vi "GyroRxLoop.vi"   [LabVIEW 2016]
uses:
  GyroRxLoopData.ctl
  GyroRxLoopStates.ctl
  GyroSBITSample.ctl
  GyroLBITSample.ctl
  GyroSample.ctl
  GyroErrorSample.ctl
  GyroErrorCodes.ctl
  <vilib>/Platform/TimedLoop/XDataNode/timing_clust.ctl
  <vilib>/Platform/TimedLoop/XDataNode/nitl_modes.ctl
  <vilib>/Platform/TimedLoop/XDataNode/wakeup.ctl
  <vilib>/rvi/Emulation/niFpgaSctlEmulationGetInTimedLoop.vi
  <vilib>/rvi/Emulation/niFpgaEmulationReportErrorSimple.vi
  <vilib>/rvi/Emulation/niFpgaGetClockAttributes.vi
  <vilib>/rvi/Emulation/niFpgaCriticalErrorInLSC.vi
  <vilib>/rvi/Emulation/niFpgaEmulationIsFPGAContextNoSignature.vi
  <vilib>/rvi/errors/niFpgaSetErrorForExecOnDevCompSimple.vi
  <vilib>/rvi/eio/common/nirviEmuReportErrorAndStop.vi
  <vilib>/rvi/DataTransferAndStorage/Container/Common/niFpgaContainerGetUniqueNameForEmu.vi
  <vilib>/rvi/FIFO/Fifo_Resource/nirvififoEmulationSetSize.vi
  <vilib>/rvi/FIFO/Fifo_Resource/nirviFifoEmulationQueueMgr.vi
  <instcachedir>/0/nirviFifoEmulationQueueMgr_E5CAEC123FF24DC58D834DCA3CDAA9B5.lvgen/nirviFifoEmulationQueueMgr_E5CAEC123FF24DC58D834DCA3CDAA9B5_009.vi
  <vilib>/Utility/error.llb/Clear Errors.vi
  <vilib>/rvi/FIFO/Fifo_Resource/nirvififoEmulationCreateLock.vi
  <vilib>/rvi/Emulation/niFpgaProcessEmulError.vi
  <vilib>/rvi/FIFO/Fifo_Resource/nirvififoEmulationObtainLock.vi
  <vilib>/rvi/FIFO/Fifo_Resource/nirvififoEmulationReleaseLock.vi
  <vilib>/rvi/occurrence/nirviWaitOnOccurrenceBase.vi
  <vilib>/rvi/errors/nirviReportUnexpectedCaseInternalError.vi
  <vilib>/rvi/errors/nirviReportUnexpectedCaseInternalError (U32).vi
  <vilib>/rvi/FIFO/Fifo_Resource/nirvififoEmulationDetermineInputValidOut.vi
  <vilib>/rvi/Memory/Memory_Emulation/niFpgaMemoryEmulationCacheClearOnFirstRun.vi
  <vilib>/rvi/Memory/Memory_Emulation/nirvimemoryEmulationManagerCache_MakeExclusive.vi
  <vilib>/rvi/Memory/Memory_Emulation/niFpgaMemoryEmulationValidateCache.vi
  <vilib>/rvi/Memory/Memory_Emulation/nirvimemoryEmulationManagerCache_InsertValue.vi
  <vilib>/rvi/Memory/Memory_Emulation/nirvimemoryEmulationManagerCache_ReleaseExclusive.vi
  <vilib>/rvi/Memory/Memory_Emulation/nirvimemoryEmulationManagerCache_GetValue.vi
  <vilib>/rvi/Memory/Memory_Emulation/nirvimemoryEmulationManagerCache_SetValue.vi
  <instcachedir>/0/nirviFifoEmulationQueueMgr_E5CAEC123FF24DC58D834DCA3CDAA9B5.lvgen/nirviFifoEmulationQueueMgr_E5CAEC123FF24DC58D834DCA3CDAA9B5_040.vi
  <instcachedir>/0/nirviFifoEmulationQueueMgr_E5CAEC123FF24DC58D834DCA3CDAA9B5.lvgen/nirviFifoEmulationQueueMgr_E5CAEC123FF24DC58D834DCA3CDAA9B5_041.vi
  <instcachedir>/0/nirviFifoEmulationQueueMgr_E5CAEC123FF24DC58D834DCA3CDAA9B5.lvgen/nirviFifoEmulationQueueMgr_E5CAEC123FF24DC58D834DCA3CDAA9B5_004.vi
  <instcachedir>/0/nirviFifoEmulationQueueMgr_E5CAEC123FF24DC58D834DCA3CDAA9B5.lvgen/nirviFifoEmulationQueueMgr_E5CAEC123FF24DC58D834DCA3CDAA9B5_006.vi
  <instcachedir>/0/nirviFifoEmulationQueueMgr_E5CAEC123FF24DC58D834DCA3CDAA9B5.lvgen/nirviFifoEmulationQueueMgr_E5CAEC123FF24DC58D834DCA3CDAA9B5_042.vi
  <instcachedir>/0/nirviFifoEmulationQueueMgr_E5CAEC123FF24DC58D834DCA3CDAA9B5.lvgen/nirviFifoEmulationQueueMgr_E5CAEC123FF24DC58D834DCA3CDAA9B5_043.vi
  <vilib>/Platform/TimedLoop/XDataNode/XDataNode.xnode
  <vilib>/rvi/DataTransferAndStorage/Container/XNode/niFpgaContainer.xnode
  <vilib>/rvi/FIFO/Fifo_Resource/nirvififoEmulationRead.vi
  <vilib>/rvi/FIFO/Fifo_Resource/nirvififoEmulationWrite.vi
  <vilib>/rvi/DataTransferAndStorage/Register/Emulation/niFpgaRegisterEmulation.vi
  <vilib>/Platform/TimedLoop/XDataNode/XDNodeRunTimeDep.lvlib
types:
  T1 = typedef "GyroRxLoopData.ctl" = cluster{"State":T2, "Timestamp":u64, "Timeout":i32, "CRC":u32, "Checksum":u8, "IsLBIT":bool, "ReservedCount":u8, "SBITSample":T3, "LBITSample":T4, "Sample":T5, "ErrorSample":T6}
  T2 = typedef "GyroRxLoopStates.ctl" = enum16{"ReadHeader3", "IgnoreASCIIResponse", "ReadNormalHeader2", "ReadNormalHeader1", "ReadBITHeader0", "ReadBIT0", "ReadBIT1", "ReadBIT2", "ReadBIT3", "ReadBIT4", "ReadBIT5", "ReadBIT6", "ReadBIT7", "ReadChecksum", "PrepareSBIT", "MoveSBIT", "PrepareLBIT", "MoveLBIT", "ReadSampleHeader0", "ReadSampleX3", "ReadSampleX2", "ReadSampleX1", "ReadSampleX0", "ReadSampleY3", "ReadSampleY2", "ReadSampleY1", "ReadSampleY0", "ReadSampleZ3", "ReadSampleZ2", "ReadSampleZ1", "ReadSampleZ0", "ReadSampleReserved", "ReadSampleStatus", "ReadSampleSequenceNumber", "ReadSampleTemperature1", "ReadSampleTemperature0", "ReadSampleCRC3", "ReadSampleCRC2", "ReadSampleCRC1", "ReadSampleCRC0", "VerifyCRC", "PrepareSample", "MoveSample", "ResponseHeaderError", "ResponseCRCError", "ResponseTimeoutError", "ResponseChecksumError", "PrepareErrorCode", "MoveErrorCode", "ClearCRC", "WaitForCRCCleared"}
  T3 = typedef "GyroSBITSample.ctl" = cluster{"Timestamp":u64, "TxBytes":u64, "RxBytes":u64, "TxFrames":u64, "RxFrames":u64, "BIT0":u8, "BIT1":u8, "BIT2":u8, "BIT3":u8, "BIT4":u8, "BIT5":u8}
  T4 = typedef "GyroLBITSample.ctl" = cluster{"Timestamp":u64, "TxBytes":u64, "RxBytes":u64, "TxFrames":u64, "RxFrames":u64, "BIT0":u8, "BIT1":u8, "BIT2":u8, "BIT3":u8, "BIT4":u8, "BIT5":u8, "BIT6":u8, "BIT7":u8}
  T5 = typedef "GyroSample.ctl" = cluster{"Timestamp":u64, "TxBytes":u64, "RxBytes":u64, "TxFrames":u64, "RxFrames":u64, "GyroX":u32, "GyroY":u32, "GyroZ":u32, "Status":u8, "SequenceNumber":u8, "Temperature":i16}
  T6 = typedef "GyroErrorSample.ctl" = cluster{"Timestamp":u64, "TxBytes":u64, "RxBytes":u64, "TxFrames":u64, "RxFrames":u64, "ErrorCode":T7}
  T7 = typedef "GyroErrorCodes.ctl" = enum8{"None", "ResponseHeaderError", "ResponseCRCError", "ResponseTimeoutError", "ResponseChecksumError"}
  T8 = typedef "XDNodeRunTimeDep.lvlib/timing_clust.ctl" = cluster{"Expected End [f-1]":u64, "Actual End [f-1]":u64, "Finished Late? [f-1]":bool, "Expected End [i-1]":u64, "Actual End [i-1]":u64, "Finished Late? [i-1]":bool, "Expected Start [i]":u64, "Actual Start [i]":u64, "Expected Start [f]":u64, "Actual Start [f]":u64, "Source Name":string, "Structure Name":string, "Period":i64, "Deadline":i64, "Offset":i64, "Start":i64, "Priority":i32, "Timeout":i32, "Mode":T9, "Wakeup Reason":T10, "Error":errorcluster, "Source Type":string, "Secondary Source Type":string, "Global End Time":u64, "Global Start Time":u64, "Frame Duration":u64, "Iteration Duration":u64, "Assigned CPU":i32, "I/O Scan Engine Mode":u32}
  T9 = typedef "XDNodeRunTimeDep.lvlib/nitl_modes.ctl" = enum32{"No Change", "Process missed periods, maintain original phase", "Discard missed periods, maintain original phase", "Process missed periods, ignore original phase", "Discard missed periods, ignore original phase"}
  T10 = typedef "XDNodeRunTimeDep.lvlib/wakeup.ctl" = enum32{"Normal", "Aborted", "Asynchronous wakeup", "Timing source error", "Timed loop error", "Timeout"}
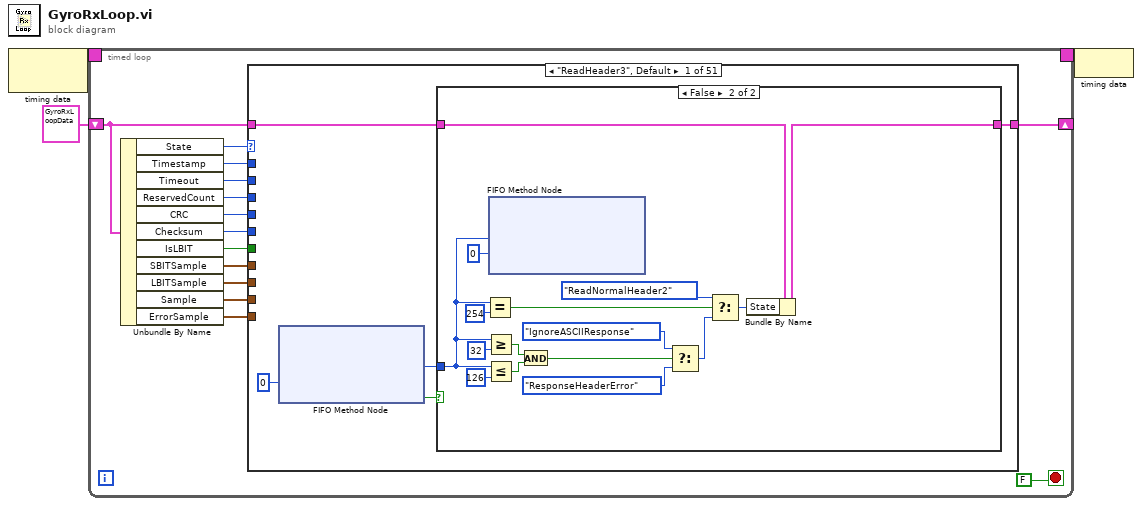
[diagram p0: block diagram]
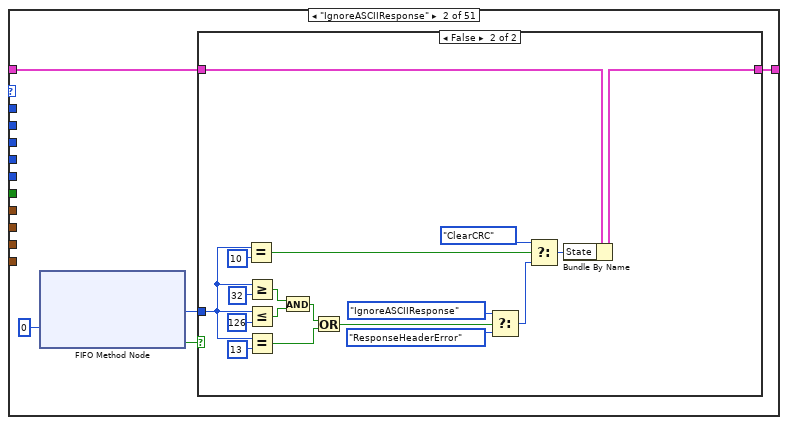
[diagram p3: hidden frame]
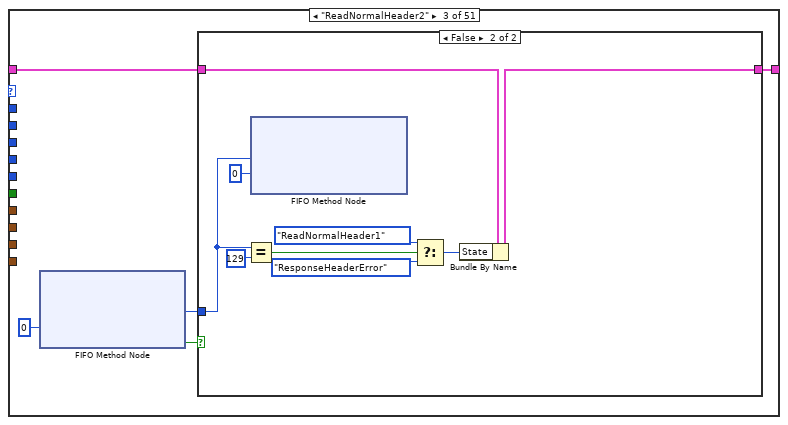
[diagram p5: hidden frame]
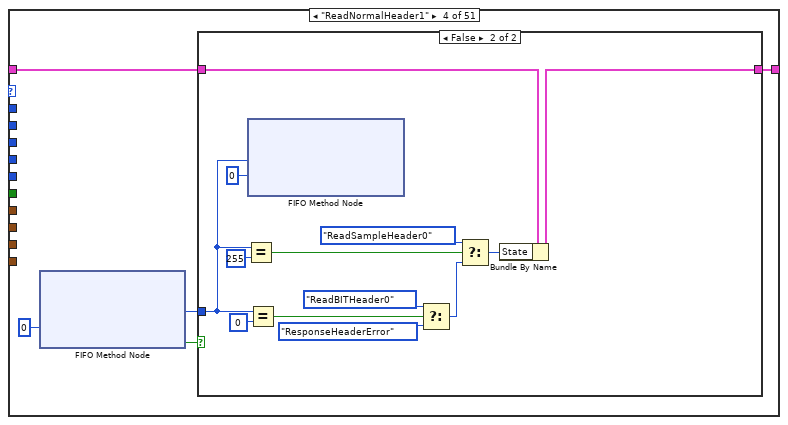
[diagram p7: hidden frame]
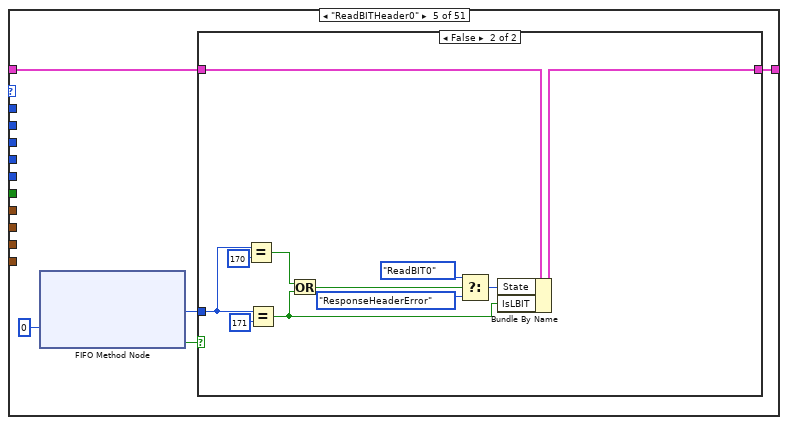
[diagram p9: hidden frame]
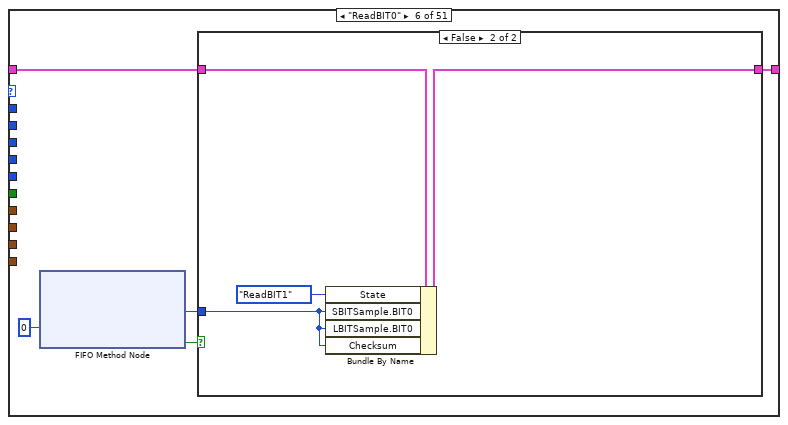
[diagram p11: hidden frame]
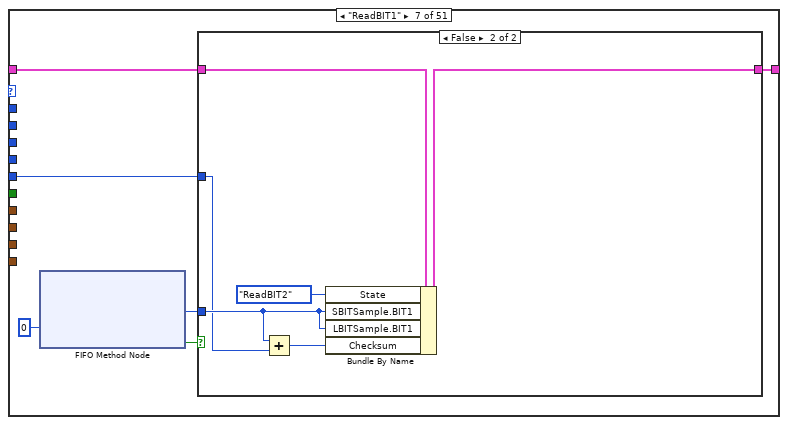
[diagram p13: hidden frame]
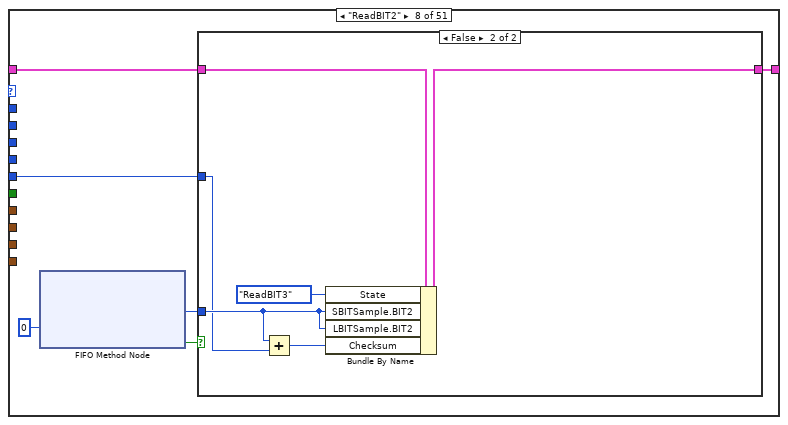
[diagram p15: hidden frame]
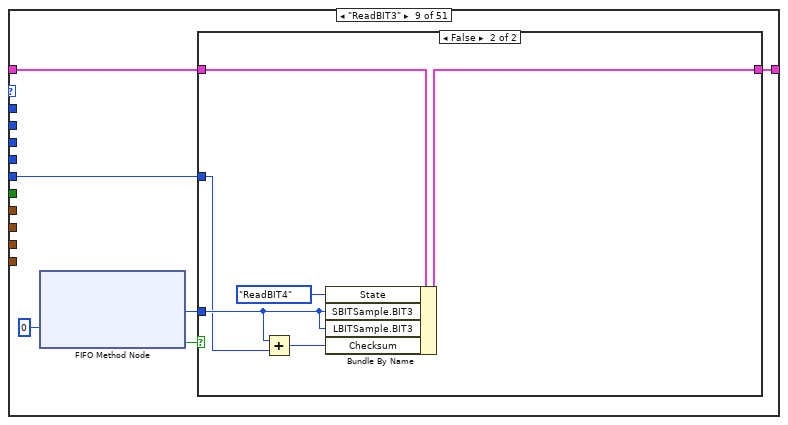
[diagram p17: hidden frame]
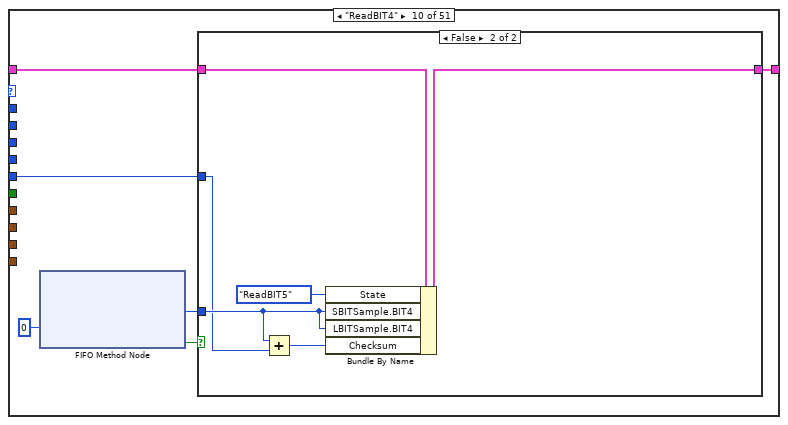
[diagram p19: hidden frame]
diagram:
  n1 = node-c288() -> (w3:T8)  [unwired: 1 in]
  n2 = timed-loop {
    timing: w3 -> [_]
    timing-out: [_] -> w2
    shift-right: [w17] -> _
    shift-left: T1 {"State"=enum."ReadHeader3", "Timestamp"=0, "Timeout"=0, "CRC"=0, "Checksum"=0, "IsLBIT"=FALSE, "ReservedCount"=0, "SBITSample"={"Timestamp"=0, "TxBytes"=0, "RxBytes"=0, "TxFrames"=0, "RxFrames"=0, "BIT0"=0, "BIT1"=0, "BIT2"=0, "BIT3"=0, "BIT4"=0, "BIT5"=0}, "LBITSample"={"Timestamp"=0, "TxBytes"=0, "RxBytes"=0, "TxFrames"=0, "RxFrames"=0, "BIT0"=0, "BIT1"=0, "BIT2"=0, "BIT3"=0, "BIT4"=0, "BIT5"=0, "BIT6"=0, "BIT7"=0}, "Sample"={"Timestamp"=0, "TxBytes"=0, "RxBytes"=0, "TxFrames"=0, "RxFrames"=0, "GyroX"=0, "GyroY"=0, "GyroZ"=0, "Status"=0, "SequenceNumber"=0, "Temperature"=0}, "ErrorSample"={"Timestamp"=0, "TxBytes"=0, "RxBytes"=0, "TxFrames"=0, "RxFrames"=0, "ErrorCode"=enum."None"}} ("GyroRxLoopData") -> [w16]
    stop <- FALSE stop-if-true
    n3 = Unbundle By Name(w16) -> ("State"=w15:T2, "Timestamp"=w14:u64, "Timeout"=w13:i32, "ReservedCount"=w9:u8, "CRC"=w12:u32, "Checksum"=w11:u8, "IsLBIT"=w10:bool, "SBITSample"=w8:T3, "LBITSample"=w7:T4, "Sample"=w6:T5, "ErrorSample"=w5:T6)
    n4 = case shown="\"ReadHeader3\", Default" w15 {
      tunnel: [w18 w40 w64 w79 w98 w115 w126 w139 w152 w165 w179 w195 w208 w222 w245 w250 w258 w263 w265 w280 w294 w310 w326 w340 w354 w370 w386 w400 w414 w430 w446 w462 w479 w490 w501 w515 w529 w545 w561 w577 w591 w611 w616 w620 w624 w628 w632 w640 w645 w650 w657] -> w17
      tunnel: w16 -> [w19 w41 w65 w80 w99 w116 w127 w140 w153 w166 w180 w196 w209 w223 w246 w251 w259 w264 w266 w281 w295 w311 w327 w341 w355 w371 w387 w401 w415 w431 w447 w463 w480 w491 w502 w516 w530 w546 w562 w578 w592 w612 w617 w621 w625 w629 w633 w641 w646 w651 w658]
      tunnel: w14 -> [_ _ _ _ _ _ _ _ _ _ _ _ _ _ w243 _ w256 _ _ _ _ _ _ _ _ _ _ _ _ _ _ _ _ _ _ _ _ _ _ _ _ w609 _ _ _ _ _ w638 _ _ _]
      tunnel: w13 -> [_ _ _ _ _ _ _ _ _ _ _ _ _ _ _ _ _ _ _ _ _ _ _ _ _ _ _ _ _ _ _ _ _ _ _ _ _ _ _ _ _ _ _ _ _ _ _ _ _ _ _]
      tunnel: w12 -> [_ _ _ _ _ _ _ _ _ _ _ _ _ _ _ _ _ _ _ _ _ _ _ _ _ _ _ _ _ _ _ _ _ _ _ _ _ w544 w560 w576 w590 _ _ _ _ _ _ _ _ _ _]
      tunnel: w11 -> [_ _ _ _ _ _ w125 w138 w151 w164 w178 w194 w207 w221 _ _ _ _ _ _ _ _ _ _ _ _ _ _ _ _ _ _ _ _ _ _ _ _ _ _ _ _ _ _ _ _ _ _ _ _ _]
      tunnel: w10 -> [_ _ _ _ _ _ _ _ _ _ w177 _ _ w220 _ _ _ _ _ _ _ _ _ _ _ _ _ _ _ _ _ _ _ _ _ _ _ _ _ _ _ _ _ _ _ _ _ _ _ _ _]
      tunnel: w9 -> [_ _ _ _ _ _ _ _ _ _ _ _ _ _ _ _ _ _ _ _ _ _ _ _ _ _ _ _ _ _ _ w461 _ _ _ _ _ _ _ _ _ _ _ _ _ _ _ _ _ _ _]
      tunnel: w8 -> [_ _ _ _ _ _ _ _ _ _ _ _ _ _ _ w247 _ _ _ _ _ _ _ _ _ _ _ _ _ _ _ _ _ _ _ _ _ _ _ _ _ _ _ _ _ _ _ _ _ _ _]
      tunnel: w7 -> [_ _ _ _ _ _ _ _ _ _ _ _ _ _ _ _ _ w260 _ _ _ _ _ _ _ _ _ _ _ _ _ _ _ _ _ _ _ _ _ _ _ _ _ _ _ _ _ _ _ _ _]
      tunnel: w6 -> [_ _ _ _ _ _ _ _ _ _ _ _ _ _ _ _ _ _ _ _ _ _ _ _ _ _ _ _ _ _ _ _ _ _ _ _ _ _ _ _ _ _ w614 _ _ _ _ _ _ _ _]
      tunnel: w5 -> [_ _ _ _ _ _ _ _ _ _ _ _ _ _ _ _ _ _ _ _ _ _ _ _ _ _ _ _ _ _ _ _ _ _ _ _ _ _ _ _ _ _ _ _ _ _ _ _ w643 _ _]
      frame "ReadHeader3", Default {
        n5 = xnode ("FIFO Method Node")("Timeout"=0) -> ("Element"=w21:u8, "Timed Out?"=w20:bool)  [unwired: 1 in, 1 out]
        n6 = case shown="False" w20 {
          tunnel: w21 -> [_ w25]
          tunnel: w19 -> [w23 w28]
          tunnel: [w23 w27] -> w18
          frame True {
          }
          frame False {
            n7 = Equal?(x=w25, y=u8 254) -> (x = y?=w29:bool)
            n8 = Greater Or Equal?(x=w25, y=u8 32) -> (x >= y?=w36:bool)
            n9 = Less Or Equal?(x=w25, y=u8 126) -> (x <= y?=w35:bool)
            n10 = xnode ("FIFO Method Node")("Element"=w25, "Timeout"=0) -> ()  [unwired: 1 in, 2 out]
            n11 = And(x=w36, y=w35) -> (x .and. y?=w34:bool)
            n12 = Select(t=GyroRxLoopStates."IgnoreASCIIResponse", s=w34, f=GyroRxLoopStates."ResponseHeaderError" ("GyroRxLoopStates")) -> (s? t:f=w33:T2)
            n13 = Select(t=GyroRxLoopStates."ReadNormalHeader2", s=w29, f=w33) -> (s? t:f=w26:T2)
            n14 = Bundle By Name(cluster=w28, "State"=w26) -> (w27:T1)
          }
        }
      }
      frame "IgnoreASCIIResponse" {
        n15 = xnode ("FIFO Method Node")("Timeout"=0) -> ("Element"=w43:u8, "Timed Out?"=w42:bool)  [unwired: 1 in, 1 out]
        n16 = case shown="False" w42 {
          tunnel: w43 -> [_ w54]
          tunnel: w41 -> [w45 w58]
          tunnel: [w45 w57] -> w40
          frame True {
          }
          frame False {
            n17 = Equal?(x=w54, y=u8 10) -> (x = y?=w59:bool)
            n18 = Greater Or Equal?(x=w54, y=u8 32) -> (x >= y?=w53:bool)
            n19 = Less Or Equal?(x=w54, y=u8 126) -> (x <= y?=w52:bool)
            n20 = Equal?(x=w54, y=u8 13) -> (x = y?=w50:bool)
            n21 = And(x=w53, y=w52) -> (x .and. y?=w51:bool)
            n22 = Or(x=w51, y=w50) -> (x .or. y?=w49:bool)
            n23 = Select(t=GyroRxLoopStates."IgnoreASCIIResponse", s=w49, f=GyroRxLoopStates."ResponseHeaderError" ("t")) -> (s? t:f=w46:T2)
            n24 = Select(t=GyroRxLoopStates."ClearCRC", s=w59, f=w46) -> (s? t:f=w56:T2)
            n25 = Bundle By Name(cluster=w58, "State"=w56) -> (w57:T1)
          }
        }
      }
      frame "ReadNormalHeader2" {
        n26 = xnode ("FIFO Method Node")("Timeout"=0) -> ("Element"=w67:u8, "Timed Out?"=w66:bool)  [unwired: 1 in, 1 out]
        n27 = case shown="False" w66 {
          tunnel: w67 -> [_ w70]
          tunnel: w65 -> [w69 w75]
          tunnel: [w69 w74] -> w64
          frame True {
          }
          frame False {
            n28 = Equal?(x=w70, y=u8 129) -> (x = y?=w76:bool)
            n29 = xnode ("FIFO Method Node")("Element"=w70, "Timeout"=0) -> ()  [unwired: 1 in, 2 out]
            n30 = Select(t=GyroRxLoopStates."ReadNormalHeader1", s=w76, f=GyroRxLoopStates."ResponseHeaderError") -> (s? t:f=w73:T2)
            n31 = Bundle By Name(cluster=w75, "State"=w73) -> (w74:T1)
          }
        }
      }
      frame "ReadNormalHeader1" {
        n32 = xnode ("FIFO Method Node")("Timeout"=0) -> ("Element"=w82:u8, "Timed Out?"=w81:bool)  [unwired: 1 in, 1 out]
        n33 = case shown="False" w81 {
          tunnel: w82 -> [_ w85]
          tunnel: w80 -> [w84 w94]
          tunnel: [w84 w93] -> w79
          frame True {
          }
          frame False {
            n34 = Equal?(x=w85, y=u8 255) -> (x = y?=w95:bool)
            n35 = xnode ("FIFO Method Node")("Element"=w85, "Timeout"=0) -> ()  [unwired: 1 in, 2 out]
            n36 = Equal?(x=w85, y=u8 0) -> (x = y?=w90:bool)
            n37 = Select(t=GyroRxLoopStates."ReadBITHeader0" ("f"), s=w90, f=GyroRxLoopStates."ResponseHeaderError") -> (s? t:f=w87:T2)
            n38 = Select(t=GyroRxLoopStates."ReadSampleHeader0", s=w95, f=w87) -> (s? t:f=w92:T2)
            n39 = Bundle By Name(cluster=w94, "State"=w92) -> (w93:T1)
          }
        }
      }
      frame "ReadBITHeader0" {
        n40 = xnode ("FIFO Method Node")("Timeout"=0) -> ("Element"=w101:u8, "Timed Out?"=w100:bool)  [unwired: 1 in, 1 out]
        n41 = case shown="False" w100 {
          tunnel: w101 -> [_ w108]
          tunnel: w99 -> [w103 w112]
          tunnel: [w103 w111] -> w98
          frame True {
          }
          frame False {
            n42 = Equal?(x=w108, y=u8 170) -> (x = y?=w107:bool)
            n43 = Equal?(x=w108, y=u8 171) -> (x = y?=w105:bool)
            n44 = Or(x=w107, y=w105) -> (x .or. y?=w106:bool)
            n45 = Select(t=GyroRxLoopStates."ReadBIT0", s=w106, f=GyroRxLoopStates."ResponseHeaderError") -> (s? t:f=w110:T2)
            n46 = Bundle By Name(cluster=w112, "State"=w110, "IsLBIT"=w105) -> (w111:T1)
          }
        }
      }
      frame "ReadBIT0" {
        n47 = xnode ("FIFO Method Node")("Timeout"=0) -> ("Element"=w118:u8, "Timed Out?"=w117:bool)  [unwired: 1 in, 1 out]
        n48 = case shown="False" w117 {
          tunnel: w118 -> [_ w121]
          tunnel: w116 -> [w120 w124]
          tunnel: [w120 w123] -> w115
          frame True {
          }
          frame False {
            n49 = Bundle By Name(cluster=w124, "State"=GyroRxLoopStates."ReadBIT1" ("t"), "SBITSample.BIT0"=w121, "LBITSample.BIT0"=w121, "Checksum"=w121) -> (w123:T1)
          }
        }
      }
      frame "ReadBIT1" {
        n50 = xnode ("FIFO Method Node")("Timeout"=0) -> ("Element"=w129:u8, "Timed Out?"=w128:bool)  [unwired: 1 in, 1 out]
        n51 = case shown="False" w128 {
          tunnel: w129 -> [_ w134]
          tunnel: w127 -> [w131 w137]
          tunnel: [w131 w136] -> w126
          tunnel: w125 -> [_ w133]
          frame True {
          }
          frame False {
            n52 = Add(x=w134, y=w133) -> (x+y=w132:u8)
            n53 = Bundle By Name(cluster=w137, "State"=GyroRxLoopStates."ReadBIT2" ("t"), "SBITSample.BIT1"=w134, "LBITSample.BIT1"=w134, "Checksum"=w132) -> (w136:T1)
          }
        }
      }
      frame "ReadBIT2" {
        n54 = xnode ("FIFO Method Node")("Timeout"=0) -> ("Element"=w142:u8, "Timed Out?"=w141:bool)  [unwired: 1 in, 1 out]
        n55 = case shown="False" w141 {
          tunnel: w142 -> [_ w147]
          tunnel: w140 -> [w144 w150]
          tunnel: [w144 w149] -> w139
          tunnel: w138 -> [_ w146]
          frame True {
          }
          frame False {
            n56 = Add(x=w147, y=w146) -> (x+y=w145:u8)
            n57 = Bundle By Name(cluster=w150, "State"=GyroRxLoopStates."ReadBIT3" ("t"), "SBITSample.BIT2"=w147, "LBITSample.BIT2"=w147, "Checksum"=w145) -> (w149:T1)
          }
        }
      }
      frame "ReadBIT3" {
        n58 = xnode ("FIFO Method Node")("Timeout"=0) -> ("Element"=w155:u8, "Timed Out?"=w154:bool)  [unwired: 1 in, 1 out]
        n59 = case shown="False" w154 {
          tunnel: w155 -> [_ w160]
          tunnel: w153 -> [w157 w163]
          tunnel: [w157 w162] -> w152
          tunnel: w151 -> [_ w159]
          frame True {
          }
          frame False {
            n60 = Add(x=w160, y=w159) -> (x+y=w158:u8)
            n61 = Bundle By Name(cluster=w163, "State"=GyroRxLoopStates."ReadBIT4" ("t"), "SBITSample.BIT3"=w160, "LBITSample.BIT3"=w160, "Checksum"=w158) -> (w162:T1)
          }
        }
      }
      frame "ReadBIT4" {
        n62 = xnode ("FIFO Method Node")("Timeout"=0) -> ("Element"=w168:u8, "Timed Out?"=w167:bool)  [unwired: 1 in, 1 out]
        n63 = case shown="False" w167 {
          tunnel: w168 -> [_ w173]
          tunnel: w166 -> [w170 w176]
          tunnel: [w170 w175] -> w165
          tunnel: w164 -> [_ w172]
          frame True {
          }
          frame False {
            n64 = Add(x=w173, y=w172) -> (x+y=w171:u8)
            n65 = Bundle By Name(cluster=w176, "State"=GyroRxLoopStates."ReadBIT5" ("t"), "SBITSample.BIT4"=w173, "LBITSample.BIT4"=w173, "Checksum"=w171) -> (w175:T1)
          }
        }
      }
      frame "ReadBIT5" {
        n66 = xnode ("FIFO Method Node")("Timeout"=0) -> ("Element"=w182:u8, "Timed Out?"=w181:bool)  [unwired: 1 in, 1 out]
        n67 = case shown="False" w181 {
          tunnel: w182 -> [_ w191]
          tunnel: w180 -> [w184 w193]
          tunnel: [w184 w192] -> w179
          tunnel: w178 -> [_ w190]
          tunnel: w177 -> [_ w188]
          frame True {
          }
          frame False {
            n68 = Add(x=w191, y=w190) -> (x+y=w189:u8)
            n69 = Select(t=GyroRxLoopStates."ReadBIT6", s=w188, f=GyroRxLoopStates."ReadChecksum") -> (s? t:f=w185:T2)
            n70 = Bundle By Name(cluster=w193, "State"=w185, "SBITSample.BIT5"=w191, "LBITSample.BIT5"=w191, "Checksum"=w189) -> (w192:T1)
          }
        }
      }
      frame "ReadBIT6" {
        n71 = xnode ("FIFO Method Node")("Timeout"=0) -> ("Element"=w198:u8, "Timed Out?"=w197:bool)  [unwired: 1 in, 1 out]
        n72 = case shown="False" w197 {
          tunnel: w198 -> [_ w204]
          tunnel: w196 -> [w200 w206]
          tunnel: [w200 w205] -> w195
          tunnel: w194 -> [_ w203]
          frame True {
          }
          frame False {
            n73 = Add(x=w204, y=w203) -> (x+y=w202:u8)
            n74 = Bundle By Name(cluster=w206, "State"=GyroRxLoopStates."ReadBIT7" ("t"), "LBITSample.BIT6"=w204, "Checksum"=w202) -> (w205:T1)
          }
        }
      }
      frame "ReadBIT7" {
        n75 = xnode ("FIFO Method Node")("Timeout"=0) -> ("Element"=w211:u8, "Timed Out?"=w210:bool)  [unwired: 1 in, 1 out]
        n76 = case shown="False" w210 {
          tunnel: w211 -> [_ w217]
          tunnel: w209 -> [w213 w219]
          tunnel: [w213 w218] -> w208
          tunnel: w207 -> [_ w216]
          frame True {
          }
          frame False {
            n77 = Add(x=w217, y=w216) -> (x+y=w215:u8)
            n78 = Bundle By Name(cluster=w219, "State"=GyroRxLoopStates."ReadChecksum" ("t"), "LBITSample.BIT7"=w217, "Checksum"=w215) -> (w218:T1)
          }
        }
      }
      frame "ReadChecksum" {
        n79 = xnode ("FIFO Method Node")("Timeout"=0) -> ("Element"=w225:u8, "Timed Out?"=w224:bool)  [unwired: 1 in, 1 out]
        n80 = case shown="False" w224 {
          tunnel: w225 -> [_ w236]
          tunnel: w223 -> [w227 w238]
          tunnel: [w227 w237] -> w222
          tunnel: w221 -> [_ w235]
          tunnel: w220 -> [_ w234]
          frame True {
          }
          frame False {
            n81 = Not Equal?(x=w235, y=w236) -> (x != y?=w231:bool)
            n82 = Select(t=GyroRxLoopStates."PrepareLBIT", s=w234, f=GyroRxLoopStates."PrepareSBIT" ("t")) -> (s? t:f=w229:T2)
            n83 = Select(t=GyroRxLoopStates."ResponseChecksumError", s=w231, f=w229) -> (s? t:f=w228:T2)
            n84 = Bundle By Name(cluster=w238, "State"=w228) -> (w237:T1)
          }
        }
      }
      frame "PrepareSBIT" {
        n85 = xnode "Register Write"() -> ("Data"=w242:u64)  [unwired: 1 in, 1 out]
        n86 = xnode "Register Write"() -> ("Data"=w241:u64)  [unwired: 1 in, 1 out]
        n87 = xnode "Register Write"() -> ("Data"=w240:u64)  [unwired: 1 in, 1 out]
        n88 = xnode "Register Write"() -> ("Data"=w239:u64)  [unwired: 1 in, 1 out]
        n89 = Bundle By Name(cluster=w246, "State"=GyroRxLoopStates."MoveSBIT", "SBITSample.Timestamp"=w243, "SBITSample.TxBytes"=w242, "SBITSample.RxBytes"=w241, "SBITSample.TxFrames"=w240, "SBITSample.RxFrames"=w239) -> (w245:T1)
      }
      frame "MoveSBIT" {
        n90 = xnode ("FIFO Method Node")("Element"=w247, "Timeout"=0) -> ()  [unwired: 1 in, 2 out]
        n91 = Bundle By Name(cluster=w251, "State"=GyroRxLoopStates."ClearCRC") -> (w250:T1)
      }
      frame "PrepareLBIT" {
        n92 = xnode "Register Read"() -> ("Data"=w255:u64)  [unwired: 1 in, 1 out]
        n93 = xnode "Register Read"() -> ("Data"=w254:u64)  [unwired: 1 in, 1 out]
        n94 = xnode "Register Read"() -> ("Data"=w253:u64)  [unwired: 1 in, 1 out]
        n95 = xnode "Register Read"() -> ("Data"=w252:u64)  [unwired: 1 in, 1 out]
        n96 = Bundle By Name(cluster=w259, "State"=GyroRxLoopStates."MoveLBIT", "LBITSample.Timestamp"=w256, "LBITSample.TxBytes"=w255, "LBITSample.RxBytes"=w254, "LBITSample.TxFrames"=w253, "LBITSample.RxFrames"=w252) -> (w258:T1)
      }
      frame "MoveLBIT" {
        n97 = xnode ("FIFO Method Node")("Element"=w260, "Timeout"=0) -> ()  [unwired: 1 in, 2 out]
        n98 = Bundle By Name(cluster=w264, "State"=GyroRxLoopStates."ClearCRC") -> (w263:T1)
      }
      frame "ReadSampleHeader0" {
        n99 = xnode ("FIFO Method Node")("Timeout"=0) -> ("Element"=w268:u8, "Timed Out?"=w267:bool)  [unwired: 1 in, 1 out]
        n100 = case shown="False" w267 {
          tunnel: w268 -> [_ w271]
          tunnel: w266 -> [w270 w277]
          tunnel: [w270 w276] -> w265
          frame True {
          }
          frame False {
            n101 = xnode ("FIFO Method Node")("Element"=w271, "Timeout"=0) -> ()  [unwired: 1 in, 2 out]
            n102 = Equal?(x=w271, y=u8 85) -> (x = y?=w273:bool)
            n103 = Select(t=GyroRxLoopStates."ReadSampleX3", s=w273, f=GyroRxLoopStates."ResponseHeaderError") -> (s? t:f=w275:T2)
            n104 = Bundle By Name(cluster=w277, "State"=w275) -> (w276:T1)
          }
        }
      }
      frame "ReadSampleX3" {
        n105 = xnode ("FIFO Method Node")("Timeout"=0) -> ("Element"=w283:u8, "Timed Out?"=w282:bool)  [unwired: 1 in, 1 out]
        n106 = case shown="False" w282 {
          tunnel: w283 -> [_ w290]
          tunnel: w281 -> [w285 w287]
          tunnel: [w285 w293] -> w280
          frame True {
          }
          frame False {
            n107 = To Unsigned Long Integer(number=w290) -> (unsigned 32bit integer=w289:u32)
            n108 = xnode ("FIFO Method Node")("Element"=w290, "Timeout"=0) -> ()  [unwired: 1 in, 2 out]
            n109 = Logical Shift(y=i16 24, x=w289) -> (x << y=w286:u32)
            n110 = Bundle By Name(cluster=w287, "State"=GyroRxLoopStates."ReadSampleX2" ("t"), "Sample.GyroX"=w286) -> (w293:T1)
          }
        }
      }
      frame "ReadSampleX2" {
        n111 = xnode ("FIFO Method Node")("Timeout"=0) -> ("Element"=w297:u8, "Timed Out?"=w296:bool)  [unwired: 1 in, 1 out]
        n112 = case shown="False" w296 {
          tunnel: w297 -> [_ w306]
          tunnel: w295 -> [w299 w303]
          tunnel: [w299 w309] -> w294
          frame True {
          }
          frame False {
            n113 = Unbundle By Name(w303) -> ("Sample.GyroX"=w302:u32)
            n114 = To Unsigned Long Integer(number=w306) -> (unsigned 32bit integer=w305:u32)
            n115 = xnode ("FIFO Method Node")("Element"=w306, "Timeout"=0) -> ()  [unwired: 1 in, 2 out]
            n116 = Logical Shift(y=i16 16, x=w305) -> (x << y=w301:u32)
            n117 = Or(x=w302, y=w301) -> (x .or. y?=w300:u32)
            n118 = Bundle By Name(cluster=w303, "State"=GyroRxLoopStates."ReadSampleX1" ("t"), "Sample.GyroX"=w300) -> (w309:T1)
          }
        }
      }
      frame "ReadSampleX1" {
        n119 = xnode ("FIFO Method Node")("Timeout"=0) -> ("Element"=w313:u8, "Timed Out?"=w312:bool)  [unwired: 1 in, 1 out]
        n120 = case shown="False" w312 {
          tunnel: w313 -> [_ w322]
          tunnel: w311 -> [w315 w319]
          tunnel: [w315 w325] -> w310
          frame True {
          }
          frame False {
            n121 = Unbundle By Name(w319) -> ("Sample.GyroX"=w318:u32)
            n122 = To Unsigned Long Integer(number=w322) -> (unsigned 32bit integer=w321:u32)
            n123 = xnode ("FIFO Method Node")("Element"=w322, "Timeout"=0) -> ()  [unwired: 1 in, 2 out]
            n124 = Logical Shift(y=i16 8, x=w321) -> (x << y=w317:u32)
            n125 = Or(x=w318, y=w317) -> (x .or. y?=w316:u32)
            n126 = Bundle By Name(cluster=w319, "State"=GyroRxLoopStates."ReadSampleX0" ("t"), "Sample.GyroX"=w316) -> (w325:T1)
          }
        }
      }
      frame "ReadSampleX0" {
        n127 = xnode ("FIFO Method Node")("Timeout"=0) -> ("Element"=w329:u8, "Timed Out?"=w328:bool)  [unwired: 1 in, 1 out]
        n128 = case shown="False" w328 {
          tunnel: w329 -> [_ w336]
          tunnel: w327 -> [w331 w335]
          tunnel: [w331 w339] -> w326
          frame True {
          }
          frame False {
            n129 = Unbundle By Name(w335) -> ("Sample.GyroX"=w334:u32)
            n130 = To Unsigned Long Integer(number=w336) -> (unsigned 32bit integer=w333:u32)
            n131 = xnode ("FIFO Method Node")("Element"=w336, "Timeout"=0) -> ()  [unwired: 1 in, 2 out]
            n132 = Or(x=w334, y=w333) -> (x .or. y?=w332:u32)
            n133 = Bundle By Name(cluster=w335, "State"=GyroRxLoopStates."ReadSampleY3" ("t"), "Sample.GyroX"=w332) -> (w339:T1)
          }
        }
      }
      frame "ReadSampleY3" {
        n134 = xnode ("FIFO Method Node")("Timeout"=0) -> ("Element"=w343:u8, "Timed Out?"=w342:bool)  [unwired: 1 in, 1 out]
        n135 = case shown="False" w342 {
          tunnel: w343 -> [_ w350]
          tunnel: w341 -> [w345 w347]
          tunnel: [w345 w353] -> w340
          frame True {
          }
          frame False {
            n136 = To Unsigned Long Integer(number=w350) -> (unsigned 32bit integer=w349:u32)
            n137 = xnode ("FIFO Method Node")("Element"=w350, "Timeout"=0) -> ()  [unwired: 1 in, 2 out]
            n138 = Logical Shift(y=i16 24, x=w349) -> (x << y=w346:u32)
            n139 = Bundle By Name(cluster=w347, "State"=GyroRxLoopStates."ReadSampleY2" ("t"), "Sample.GyroY"=w346) -> (w353:T1)
          }
        }
      }
      frame "ReadSampleY2" {
        n140 = xnode ("FIFO Method Node")("Timeout"=0) -> ("Element"=w357:u8, "Timed Out?"=w356:bool)  [unwired: 1 in, 1 out]
        n141 = case shown="False" w356 {
          tunnel: w357 -> [_ w366]
          tunnel: w355 -> [w359 w363]
          tunnel: [w359 w369] -> w354
          frame True {
          }
          frame False {
            n142 = Unbundle By Name(w363) -> ("Sample.GyroY"=w362:u32)
            n143 = To Unsigned Long Integer(number=w366) -> (unsigned 32bit integer=w365:u32)
            n144 = xnode ("FIFO Method Node")("Element"=w366, "Timeout"=0) -> ()  [unwired: 1 in, 2 out]
            n145 = Logical Shift(y=i16 16, x=w365) -> (x << y=w361:u32)
            n146 = Or(x=w362, y=w361) -> (x .or. y?=w360:u32)
            n147 = Bundle By Name(cluster=w363, "State"=GyroRxLoopStates."ReadSampleY1" ("t"), "Sample.GyroY"=w360) -> (w369:T1)
          }
        }
      }
      frame "ReadSampleY1" {
        n148 = xnode ("FIFO Method Node")("Timeout"=0) -> ("Element"=w373:u8, "Timed Out?"=w372:bool)  [unwired: 1 in, 1 out]
        n149 = case shown="False" w372 {
          tunnel: w373 -> [_ w382]
          tunnel: w371 -> [w375 w379]
          tunnel: [w375 w385] -> w370
          frame True {
          }
          frame False {
            n150 = Unbundle By Name(w379) -> ("Sample.GyroY"=w378:u32)
            n151 = To Unsigned Long Integer(number=w382) -> (unsigned 32bit integer=w381:u32)
            n152 = xnode ("FIFO Method Node")("Element"=w382, "Timeout"=0) -> ()  [unwired: 1 in, 2 out]
            n153 = Logical Shift(y=i16 8, x=w381) -> (x << y=w377:u32)
            n154 = Or(x=w378, y=w377) -> (x .or. y?=w376:u32)
            n155 = Bundle By Name(cluster=w379, "State"=GyroRxLoopStates."ReadSampleY0" ("t"), "Sample.GyroY"=w376) -> (w385:T1)
          }
        }
      }
      frame "ReadSampleY0" {
        n156 = xnode ("FIFO Method Node")("Timeout"=0) -> ("Element"=w389:u8, "Timed Out?"=w388:bool)  [unwired: 1 in, 1 out]
        n157 = case shown="False" w388 {
          tunnel: w389 -> [_ w396]
          tunnel: w387 -> [w391 w395]
          tunnel: [w391 w399] -> w386
          frame True {
          }
          frame False {
            n158 = Unbundle By Name(w395) -> ("Sample.GyroY"=w394:u32)
            n159 = To Unsigned Long Integer(number=w396) -> (unsigned 32bit integer=w393:u32)
            n160 = xnode ("FIFO Method Node")("Element"=w396, "Timeout"=0) -> ()  [unwired: 1 in, 2 out]
            n161 = Or(x=w394, y=w393) -> (x .or. y?=w392:u32)
            n162 = Bundle By Name(cluster=w395, "State"=GyroRxLoopStates."ReadSampleZ3" ("t"), "Sample.GyroY"=w392) -> (w399:T1)
          }
        }
      }
      frame "ReadSampleZ3" {
        n163 = xnode ("FIFO Method Node")("Timeout"=0) -> ("Element"=w403:u8, "Timed Out?"=w402:bool)  [unwired: 1 in, 1 out]
        n164 = case shown="False" w402 {
          tunnel: w403 -> [_ w410]
          tunnel: w401 -> [w405 w407]
          tunnel: [w405 w413] -> w400
          frame True {
          }
          frame False {
            n165 = To Unsigned Long Integer(number=w410) -> (unsigned 32bit integer=w409:u32)
            n166 = xnode ("FIFO Method Node")("Element"=w410, "Timeout"=0) -> ()  [unwired: 1 in, 2 out]
            n167 = Logical Shift(y=i16 24, x=w409) -> (x << y=w406:u32)
            n168 = Bundle By Name(cluster=w407, "State"=GyroRxLoopStates."ReadSampleZ2" ("t"), "Sample.GyroZ"=w406) -> (w413:T1)
          }
        }
      }
      frame "ReadSampleZ2" {
        n169 = xnode ("FIFO Method Node")("Timeout"=0) -> ("Element"=w417:u8, "Timed Out?"=w416:bool)  [unwired: 1 in, 1 out]
        n170 = case shown="False" w416 {
          tunnel: w417 -> [_ w426]
          tunnel: w415 -> [w419 w423]
          tunnel: [w419 w429] -> w414
          frame True {
          }
          frame False {
            n171 = Unbundle By Name(w423) -> ("Sample.GyroZ"=w422:u32)
            n172 = To Unsigned Long Integer(number=w426) -> (unsigned 32bit integer=w425:u32)
            n173 = xnode ("FIFO Method Node")("Element"=w426, "Timeout"=0) -> ()  [unwired: 1 in, 2 out]
            n174 = Logical Shift(y=i16 16, x=w425) -> (x << y=w421:u32)
            n175 = Or(x=w422, y=w421) -> (x .or. y?=w420:u32)
            n176 = Bundle By Name(cluster=w423, "State"=GyroRxLoopStates."ReadSampleZ1" ("t"), "Sample.GyroZ"=w420) -> (w429:T1)
          }
        }
      }
      frame "ReadSampleZ1" {
        n177 = xnode ("FIFO Method Node")("Timeout"=0) -> ("Element"=w433:u8, "Timed Out?"=w432:bool)  [unwired: 1 in, 1 out]
        n178 = case shown="False" w432 {
          tunnel: w433 -> [_ w442]
          tunnel: w431 -> [w435 w439]
          tunnel: [w435 w445] -> w430
          frame True {
          }
          frame False {
            n179 = Unbundle By Name(w439) -> ("Sample.GyroZ"=w438:u32)
            n180 = To Unsigned Long Integer(number=w442) -> (unsigned 32bit integer=w441:u32)
            n181 = xnode ("FIFO Method Node")("Element"=w442, "Timeout"=0) -> ()  [unwired: 1 in, 2 out]
            n182 = Logical Shift(y=i16 8, x=w441) -> (x << y=w437:u32)
            n183 = Or(x=w438, y=w437) -> (x .or. y?=w436:u32)
            n184 = Bundle By Name(cluster=w439, "State"=GyroRxLoopStates."ReadSampleZ0" ("t"), "Sample.GyroZ"=w436) -> (w445:T1)
          }
        }
      }
      frame "ReadSampleZ0" {
        n185 = xnode ("FIFO Method Node")("Timeout"=0) -> ("Element"=w449:u8, "Timed Out?"=w448:bool)  [unwired: 1 in, 1 out]
        n186 = case shown="False" w448 {
          tunnel: w449 -> [_ w457]
          tunnel: w447 -> [w451 w456]
          tunnel: [w451 w460] -> w446
          frame True {
          }
          frame False {
            n187 = Unbundle By Name(w456) -> ("Sample.GyroZ"=w455:u32)
            n188 = To Unsigned Long Integer(number=w457) -> (unsigned 32bit integer=w454:u32)
            n189 = xnode ("FIFO Method Node")("Element"=w457, "Timeout"=0) -> ()  [unwired: 1 in, 2 out]
            n190 = Or(x=w455, y=w454) -> (x .or. y?=w453:u32)
            n191 = Bundle By Name(cluster=w456, "State"=GyroRxLoopStates."ReadSampleReserved" ("t"), "Sample.GyroZ"=w453, "ReservedCount"=u8 0) -> (w460:T1)
          }
        }
      }
      frame "ReadSampleReserved" {
        n192 = xnode ("FIFO Method Node")("Timeout"=0) -> ("Element"=w465:u8, "Timed Out?"=w464:bool)  [unwired: 1 in, 1 out]
        n193 = case shown="False" w464 {
          tunnel: w465 -> [_ w476]
          tunnel: w463 -> [w467 w475]
          tunnel: [w467 w478] -> w462
          tunnel: w461 -> [_ w474]
          frame True {
          }
          frame False {
            n194 = Increment(x=w474) -> (x+1=w473:u8)
            n195 = xnode ("FIFO Method Node")("Element"=w476, "Timeout"=0) -> ()  [unwired: 1 in, 2 out]
            n196 = Less?(x=w473, y=u8 12) -> (x < y?=w469:bool)
            n197 = Select(t=GyroRxLoopStates."ReadSampleReserved", s=w469, f=GyroRxLoopStates."ReadSampleStatus") -> (s? t:f=w470:T2)
            n198 = Bundle By Name(cluster=w475, "State"=w470, "ReservedCount"=w473) -> (w478:T1)
          }
        }
      }
      frame "ReadSampleStatus" {
        n199 = xnode ("FIFO Method Node")("Timeout"=0) -> ("Element"=w482:u8, "Timed Out?"=w481:bool)  [unwired: 1 in, 1 out]
        n200 = case shown="False" w481 {
          tunnel: w482 -> [_ w485]
          tunnel: w480 -> [w484 w487]
          tunnel: [w484 w489] -> w479
          frame True {
          }
          frame False {
            n201 = xnode ("FIFO Method Node")("Element"=w485, "Timeout"=0) -> ()  [unwired: 1 in, 2 out]
            n202 = Bundle By Name(cluster=w487, "State"=GyroRxLoopStates."ReadSampleSequenceNumber" ("t"), "Sample.Status"=w485) -> (w489:T1)
          }
        }
      }
      frame "ReadSampleSequenceNumber" {
        n203 = xnode ("FIFO Method Node")("Timeout"=0) -> ("Element"=w493:u8, "Timed Out?"=w492:bool)  [unwired: 1 in, 1 out]
        n204 = case shown="False" w492 {
          tunnel: w493 -> [_ w496]
          tunnel: w491 -> [w495 w498]
          tunnel: [w495 w500] -> w490
          frame True {
          }
          frame False {
            n205 = xnode ("FIFO Method Node")("Element"=w496, "Timeout"=0) -> ()  [unwired: 1 in, 2 out]
            n206 = Bundle By Name(cluster=w498, "State"=GyroRxLoopStates."ReadSampleTemperature1" ("t"), "Sample.SequenceNumber"=w496) -> (w500:T1)
          }
        }
      }
      frame "ReadSampleTemperature1" {
        n207 = xnode ("FIFO Method Node")("Timeout"=0) -> ("Element"=w504:u8, "Timed Out?"=w503:bool)  [unwired: 1 in, 1 out]
        n208 = case shown="False" w503 {
          tunnel: w504 -> [_ w511]
          tunnel: w502 -> [w506 w508]
          tunnel: [w506 w514] -> w501
          frame True {
          }
          frame False {
            n209 = To Word Integer(number=w511) -> (16bit integer=w510:i16)
            n210 = xnode ("FIFO Method Node")("Element"=w511, "Timeout"=0) -> ()  [unwired: 1 in, 2 out]
            n211 = Logical Shift(y=i16 8, x=w510) -> (x << y=w507:i16)
            n212 = Bundle By Name(cluster=w508, "State"=GyroRxLoopStates."ReadSampleTemperature0" ("t"), "Sample.Temperature"=w507) -> (w514:T1)
          }
        }
      }
      frame "ReadSampleTemperature0" {
        n213 = xnode ("FIFO Method Node")("Timeout"=0) -> ("Element"=w518:u8, "Timed Out?"=w517:bool)  [unwired: 1 in, 1 out]
        n214 = case shown="False" w517 {
          tunnel: w518 -> [_ w525]
          tunnel: w516 -> [w520 w524]
          tunnel: [w520 w528] -> w515
          frame True {
          }
          frame False {
            n215 = Unbundle By Name(w524) -> ("Sample.Temperature"=w523:i16)
            n216 = To Word Integer(number=w525) -> (16bit integer=w522:i16)
            n217 = xnode ("FIFO Method Node")("Element"=w525, "Timeout"=0) -> ()  [unwired: 1 in, 2 out]
            n218 = Or(x=w523, y=w522) -> (x .or. y?=w521:i16)
            n219 = Bundle By Name(cluster=w524, "State"=GyroRxLoopStates."ReadSampleCRC3" ("t"), "Sample.Temperature"=w521) -> (w528:T1)
          }
        }
      }
      frame "ReadSampleCRC3" {
        n220 = xnode ("FIFO Method Node")("Timeout"=0) -> ("Element"=w532:u8, "Timed Out?"=w531:bool)  [unwired: 1 in, 1 out]
        n221 = case shown="False" w531 {
          tunnel: w532 -> [_ w541]
          tunnel: w530 -> [w534 w538]
          tunnel: [w534 w543] -> w529
          frame True {
          }
          frame False {
            n222 = To Unsigned Long Integer(number=w541) -> (unsigned 32bit integer=w540:u32)
            n223 = xnode ("FIFO Method Node")("Element"=TRUE, "Timeout"=0) -> ()  [unwired: 1 in, 2 out]
            n224 = Logical Shift(y=i16 24, x=w540) -> (x << y=w537:u32)
            n225 = Bundle By Name(cluster=w538, "State"=GyroRxLoopStates."ReadSampleCRC2" ("t"), "CRC"=w537) -> (w543:T1)
          }
        }
      }
      frame "ReadSampleCRC2" {
        n226 = xnode ("FIFO Method Node")("Timeout"=0) -> ("Element"=w548:u8, "Timed Out?"=w547:bool)  [unwired: 1 in, 1 out]
        n227 = case shown="False" w547 {
          tunnel: w548 -> [_ w557]
          tunnel: w546 -> [w550 w556]
          tunnel: [w550 w559] -> w545
          tunnel: w544 -> [_ w554]
          frame True {
          }
          frame False {
            n228 = To Unsigned Long Integer(number=w557) -> (unsigned 32bit integer=w553:u32)
            n229 = Logical Shift(y=i16 16, x=w553) -> (x << y=w551:u32)
            n230 = Or(x=w554, y=w551) -> (x .or. y?=w555:u32)
            n231 = Bundle By Name(cluster=w556, "State"=GyroRxLoopStates."ReadSampleCRC1" ("t"), "CRC"=w555) -> (w559:T1)
          }
        }
      }
      frame "ReadSampleCRC1" {
        n232 = xnode ("FIFO Method Node")("Timeout"=0) -> ("Element"=w564:u8, "Timed Out?"=w563:bool)  [unwired: 1 in, 1 out]
        n233 = case shown="False" w563 {
          tunnel: w564 -> [_ w573]
          tunnel: w562 -> [w566 w572]
          tunnel: [w566 w575] -> w561
          tunnel: w560 -> [_ w570]
          frame True {
          }
          frame False {
            n234 = To Unsigned Long Integer(number=w573) -> (unsigned 32bit integer=w569:u32)
            n235 = Logical Shift(y=i16 8, x=w569) -> (x << y=w567:u32)
            n236 = Or(x=w570, y=w567) -> (x .or. y?=w571:u32)
            n237 = Bundle By Name(cluster=w572, "State"=GyroRxLoopStates."ReadSampleCRC0" ("t"), "CRC"=w571) -> (w575:T1)
          }
        }
      }
      frame "ReadSampleCRC0" {
        n238 = xnode ("FIFO Method Node")("Timeout"=0) -> ("Element"=w580:u8, "Timed Out?"=w579:bool)  [unwired: 1 in, 1 out]
        n239 = case shown="False" w579 {
          tunnel: w580 -> [_ w587]
          tunnel: w578 -> [w582 w586]
          tunnel: [w582 w589] -> w577
          tunnel: w576 -> [_ w584]
          frame True {
          }
          frame False {
            n240 = To Unsigned Long Integer(number=w587) -> (unsigned 32bit integer=w583:u32)
            n241 = Or(x=w584, y=w583) -> (x .or. y?=w585:u32)
            n242 = Bundle By Name(cluster=w586, "State"=GyroRxLoopStates."VerifyCRC" ("t"), "CRC"=w585) -> (w589:T1)
          }
        }
      }
      frame "VerifyCRC" {
        n243 = xnode ("FIFO Method Node")("Timeout"=0) -> ("Element"=w594:u32, "Timed Out?"=w593:bool)  [unwired: 1 in, 1 out]
        n244 = case shown="False" w593 {
          tunnel: w594 -> [_ w601]
          tunnel: w592 -> [w596 w603]
          tunnel: [w596 w604] -> w591
          tunnel: w590 -> [_ w602]
          frame True {
          }
          frame False {
            n245 = Equal?(x=w602, y=w601) -> (x = y?=w599:bool)
            n246 = Select(t=GyroRxLoopStates."PrepareSample", s=w599, f=GyroRxLoopStates."ResponseCRCError" ("t")) -> (s? t:f=w597:T2)
            n247 = Bundle By Name(cluster=w603, "State"=w597) -> (w604:T1)
          }
        }
      }
      frame "PrepareSample" {
        n248 = xnode "Register Read"() -> ("Data"=w608:u64)  [unwired: 1 in, 1 out]
        n249 = xnode "Register Read"() -> ("Data"=w607:u64)  [unwired: 1 in, 1 out]
        n250 = xnode "Register Read"() -> ("Data"=w606:u64)  [unwired: 1 in, 1 out]
        n251 = xnode "Register Read"() -> ("Data"=w605:u64)  [unwired: 1 in, 1 out]
        n252 = Bundle By Name(cluster=w612, "State"=GyroRxLoopStates."MoveSample", "Sample.Timestamp"=w609, "Sample.TxBytes"=w608, "Sample.RxBytes"=w607, "Sample.TxFrames"=w606, "Sample.RxFrames"=w605) -> (w611:T1)
      }
      frame "MoveSample" {
        n253 = xnode ("FIFO Method Node")("Element"=w614, "Timeout"=0) -> ()  [unwired: 1 in, 2 out]
        n254 = Bundle By Name(cluster=w617, "State"=GyroRxLoopStates."ClearCRC") -> (w616:T1)
      }
      frame "ResponseHeaderError" {
        n255 = Bundle By Name(cluster=w621, "State"=GyroRxLoopStates."PrepareErrorCode", "ErrorSample.ErrorCode"=GyroErrorCodes."ResponseHeaderError" ("GyroErrorCodes")) -> (w620:T1)
      }
      frame "ResponseCRCError" {
        n256 = Bundle By Name(cluster=w625, "State"=GyroRxLoopStates."PrepareErrorCode", "ErrorSample.ErrorCode"=GyroErrorCodes."ResponseCRCError" ("GyroErrorCodes")) -> (w624:T1)
      }
      frame "ResponseTimeoutError" {
        n257 = Bundle By Name(cluster=w629, "State"=GyroRxLoopStates."PrepareErrorCode", "ErrorSample.ErrorCode"=GyroErrorCodes."ResponseTimeoutError" ("GyroErrorCodes")) -> (w628:T1)
      }
      frame "ResponseChecksumError" {
        n258 = Bundle By Name(cluster=w633, "State"=GyroRxLoopStates."PrepareErrorCode", "ErrorSample.ErrorCode"=GyroErrorCodes."ResponseChecksumError" ("GyroErrorCodes")) -> (w632:T1)
      }
      frame "PrepareErrorCode" {
        n259 = xnode "Register Read"() -> ("Data"=w637:u64)  [unwired: 1 in, 1 out]
        n260 = xnode "Register Read"() -> ("Data"=w636:u64)  [unwired: 1 in, 1 out]
        n261 = xnode "Register Read"() -> ("Data"=w635:u64)  [unwired: 1 in, 1 out]
        n262 = xnode "Register Read"() -> ("Data"=w634:u64)  [unwired: 1 in, 1 out]
        n263 = Bundle By Name(cluster=w641, "State"=GyroRxLoopStates."MoveErrorCode", "ErrorSample.Timestamp"=w638, "ErrorSample.TxBytes"=w637, "ErrorSample.RxBytes"=w636, "ErrorSample.TxFrames"=w635, "ErrorSample.RxFrames"=w634) -> (w640:T1)
      }
      frame "MoveErrorCode" {
        n264 = xnode ("FIFO Method Node")("Element"=w643, "Timeout"=0) -> ()  [unwired: 1 in, 2 out]
        n265 = Bundle By Name(cluster=w646, "State"=GyroRxLoopStates."ClearCRC") -> (w645:T1)
      }
      frame "ClearCRC" {
        n266 = xnode ("FIFO Method Node")("Element"=TRUE, "Timeout"=0) -> ()  [unwired: 1 in, 2 out]
        n267 = Bundle By Name(cluster=w651, "State"=GyroRxLoopStates."WaitForCRCCleared") -> (w650:T1)
      }
      frame "WaitForCRCCleared" {
        n268 = xnode ("FIFO Method Node")("Timeout"=0) -> ("Timed Out?"=w655:bool)  [unwired: 1 in, 2 out]
        n269 = Select(t=GyroRxLoopStates."WaitForCRCCleared", s=w655, f=GyroRxLoopStates."ReadHeader3" ("State")) -> (s? t:f=w652:T2)
        n270 = Bundle By Name(cluster=w658, "State"=w652) -> (w657:T1)
      }
    }
  }
  n271 = node-c288(w2) -> ()
